vi "Configure BERT Synchronization.vi"(8 "error in (no error)":errorcluster, 9 "Resynchronization Threshold Limit (0.4)":dbl=0.4, 10 "Enable Resynchronization (T: Enable)":bool=TRUE, 11 "VISA resource name":refnum<visa-resource-name>) -> (0 "error out":errorcluster, 3 "VISA resource name out":refnum<visa-resource-name>)   [LabVIEW 2018, in "Agilent PSG MXG Series.lvlib"]
doc: "Configures the resynchronization function.\n\n<b>Note:</b>\nIt is applicable for N5172B/82B with <b>Option UN7</b> only."
uses:
  Agilent PSG MXG Series.lvlib
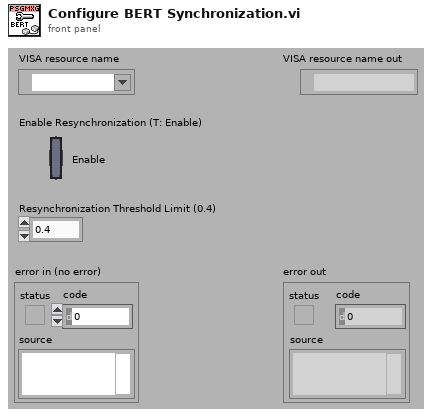
[diagram p1: front panel]
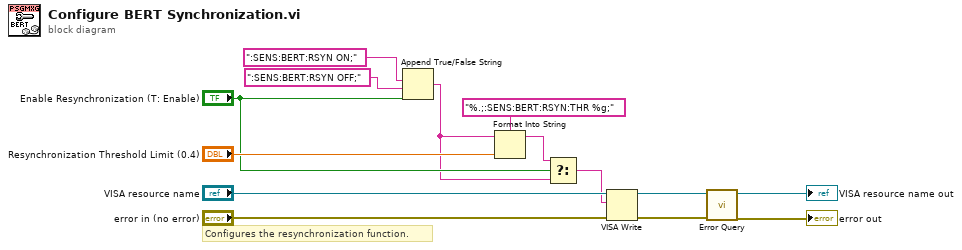
[diagram p0: block diagram]
diagram:
  # "Configures the resynchronization function."
  n1 = Append True/False String(1:"Enable Resynchronization (T: Enable)", 2:":SENS:BERT:RSYN OFF;", 3:":SENS:BERT:RSYN ON;") -> (0:w1:string)  [unwired: 1 in]
  n2 = Format Into String(format string="%.;:SENS:BERT:RSYN:THR %g;", initial string=w1, "Resynchronization Threshold Limit (0.4)") -> (resulting string=w2:string)  [unwired: 1 in, 1 out]
  n3 = Select(t=w2, s="Enable Resynchronization (T: Enable)", f=w1) -> (s? t:f=w3:string)
  n4 = VISA Write(VISA resource name="VISA resource name", write buffer=w3, error in (no error)="error in (no error)") -> (VISA resource name out=w8:refnum<visa-resource-name>, error out=w7:errorcluster)  [unwired: 1 out]
  n5 = call "Error Query.vi"("error in (no error)"=w7, "VISA resource name"=w8) -> ("error out"=→"error out":errorcluster, "VISA resource name out"=→"VISA resource name out":refnum<visa-resource-name>)  [unwired: 6 in, 2 out]
